vi "Connection Callback.vi"(7 "Owner":refnum<class>, 10 "Connection State":T1, 11 "Endpoint":refnum<class "Endpoint.lvclass">) -> ()   [LabVIEW 2020, in "LV Chat Client.lvclass"]
uses:
  LV Chat Client.lvclass
  <vilib>/IlluminatedG/lv-stream/Connection State.ctl
  <vilib>/IlluminatedG/lv-msg-simple/Stream-Simple-Msg/Endpoint/Endpoint.lvclass
  LV Chat Client.lvclass/LV Chat Client.ctl
  <vilib>/IlluminatedG/lv-stream/Stream.lvlib
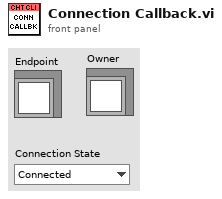
[diagram p1: front panel]
types:
  T1 = typedef "Stream.lvlib/Connection State.ctl" = enum16{"Connected", "Disconnected"}
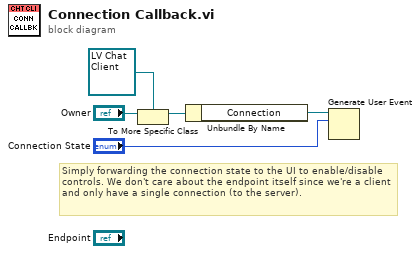
[diagram p0: block diagram]
diagram:
  # "Simply forwarding the connection state to the UI to enable/disable controls. We don't care about the endpoint itself since we're a client and only have a single connection (to the server)."
  n1 = To More Specific Class(target class=refnum<class "LV Chat Client.lvclass"> refnum ("LV Chat Client.lvclass"), reference="Owner") -> (specific class reference=w3:refnum<class "LV Chat Client.lvclass">)  [unwired: 1 in, 1 out]
  n2 = Unbundle By Name(w3) -> ("Connection"=w2:refnum<user-event>)
  n3 = Generate User Event(user event=w2, event data cluster="Connection State") -> ()  [unwired: 2 in, 2 out]
